vi "Resize.vi"(10 "Capacity":u32, 11 "TypedCircularBuffer in":refnum<class "RotateCircularBuffer.lvclass">) -> (3 "TypedCircularBuffer out":refnum<class "RotateCircularBuffer.lvclass">)   [LabVIEW 2024, in "RotateCircularBuffer.lvclass"]
uses:
  RotateCircularBuffer.lvclass
  RotateCircularBuffer.lvclass/RotateCircularBuffer.ctl
  Type.ctl
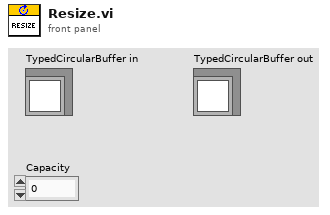
[diagram p1: front panel]
types:
  T1 = typedef "RotateCircularBuffer.lvclass/Type.ctl" = u8
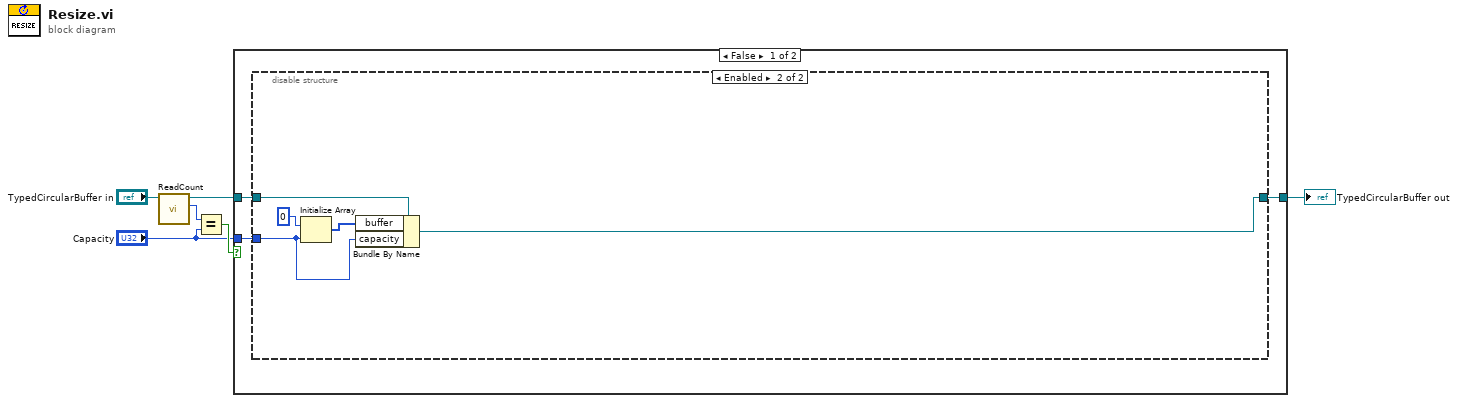
[diagram p0: block diagram]
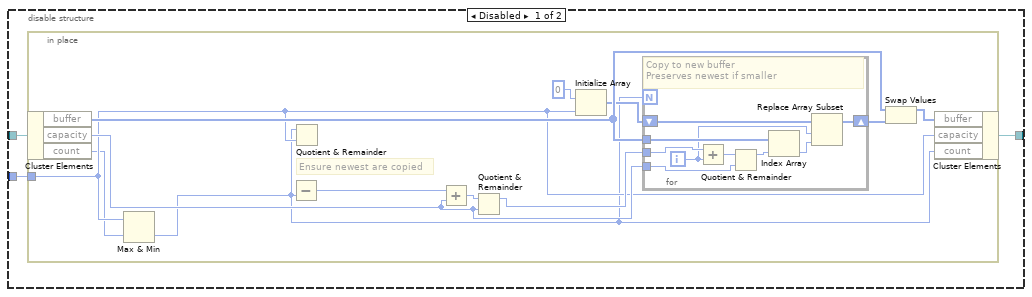
[diagram p2: hidden frame]
diagram:
  n1 = call "ReadCount.vi"("TypedCircularBuffer in"="TypedCircularBuffer in") -> ("size"=w5:u32, "TypedCircularBuffer out"=w2:refnum<class "RotateCircularBuffer.lvclass">)  [unwired: 9 in]
  n2 = Equal?(x=w5, y="Capacity") -> (x = y?=w4:bool)
  n3 = case shown="False" w4 {
    tunnel: [w7 w39] -> w3
    tunnel: w2 -> [w9 w39]
    tunnel: "Capacity" -> [w8 _]
    frame False {
      n4 = disable-structure shown="Enabled" {
        disable-tunnel: w9 -> [w12 w37]
        disable-tunnel: w8 -> [w11 w34]
        disable-tunnel: [w10 w38] -> w7
        frame Disabled {
          n5 = in-place {
            in-place-border: w11 -> [w15]
            # "Ensure newest are copied"
            n6 = in-place-cluster #1(w12) -> ("buffer"=w23:T1[], "capacity"=w18:u32, "count"=w14:u32)
            n7 = Max & Min(x=w15, y=w14) -> (min(x,y)=w13:u32)  [unwired: 1 out]
            n8 = Subtract(y=w13) -> (x-y=w20:u32)  [unwired: 1 in]
            n9 = Quotient & Remainder(x=w13, y=w15) -> ()  [unwired: 2 out]
            n10 = Add(x=w20, y=w18) -> (x+y=w19:u32)
            n11 = Quotient & Remainder(x=w19, y=w18) -> (x-y*floor(x/y)=w17:u32)  [unwired: 1 out]
            n12 = Initialize Array(T1 0 ("Type"), w15) -> (w21:T1[])
            n13 = for {
              N: w13 -> [_]
              tunnel: w23 -> [w33]
              tunnel: w17 -> [w32]
              tunnel: w18 -> [w30]
              shift-right: [w28] -> w16
              shift-left: w21 -> [w29]
              i -> [w26]
              # "Copy to new buffer\nPreserves newest if smaller"
              n14 = Add(x=w32, y=w26) -> (x+y=w31:u32)
              n15 = Quotient & Remainder(x=w31, y=w30) -> (x-y*floor(x/y)=w27:u32)  [unwired: 1 out]
              n16 = Index Array(array=w33, index=w27) -> (element=w25:T1)
              n17 = Replace Array Subset(array=w29, new element=w25, index=w26) -> (w28:T1[])
            }
            n18 = Swap Values(12:w23, 14:w16) -> (1:w22:T1[])  [unwired: 1 in, 1 out]
            n19 = in-place-cluster #1("buffer"=w22, "capacity"=w15, "count"=w13) -> (w10:refnum<class "RotateCircularBuffer.lvclass">)
          }
        }
        frame Enabled {
          n20 = Initialize Array(T1 0 ("Type"), w34) -> (w35:T1[])
          n21 = Bundle By Name(cluster=w37, "buffer"=w35, "capacity"=w34) -> (w38:refnum<class "RotateCircularBuffer.lvclass">)
        }
      }
    }
    frame True {
    }
  }
  "TypedCircularBuffer out" <- w3
